vi "Merge Frequency Arrays.vi"(10 "New Frequencies to merge":dbl[](array[numeric]), 11 "Statistics Data":T1) -> (3 "Statistics Data 2":T1)   [LabVIEW 2011]
uses:
  Statistics Data.ctl
  CGI SimpleStat Results.ctl
panel:
  out "Array":dbl[](array[numeric]) format="%_17f"
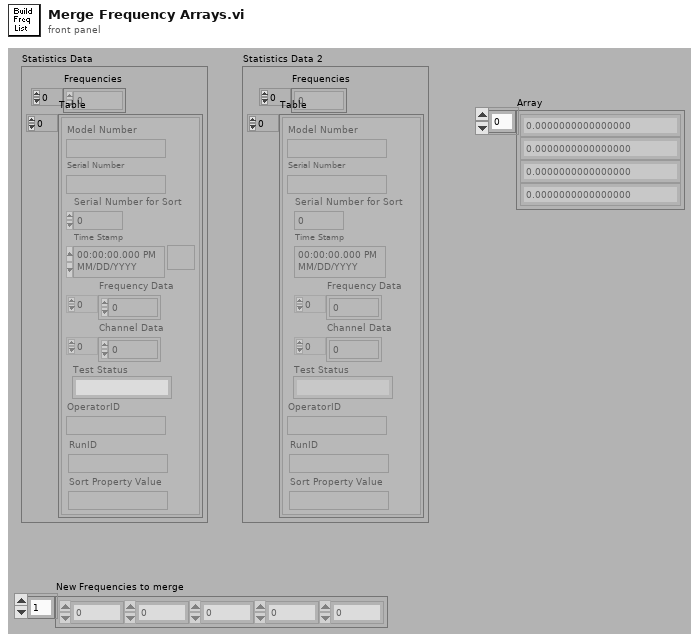
[diagram p1: front panel]
types:
  T1 = typedef "Statistics Data.ctl" = cluster{"Table":T2[], "Frequencies":dbl[]}
  T2 = typedef "CGI SimpleStat Results.ctl" = cluster{"Model Number":string, "Serial Number for Sort":i32, "Serial Number":string, "Time Stamp":timestamp, "Channel Data":dbl[], "Test Status":string, "OperatorID":string, "Frequency Data":dbl[], "RunID":string, "Sort Property Value":string}
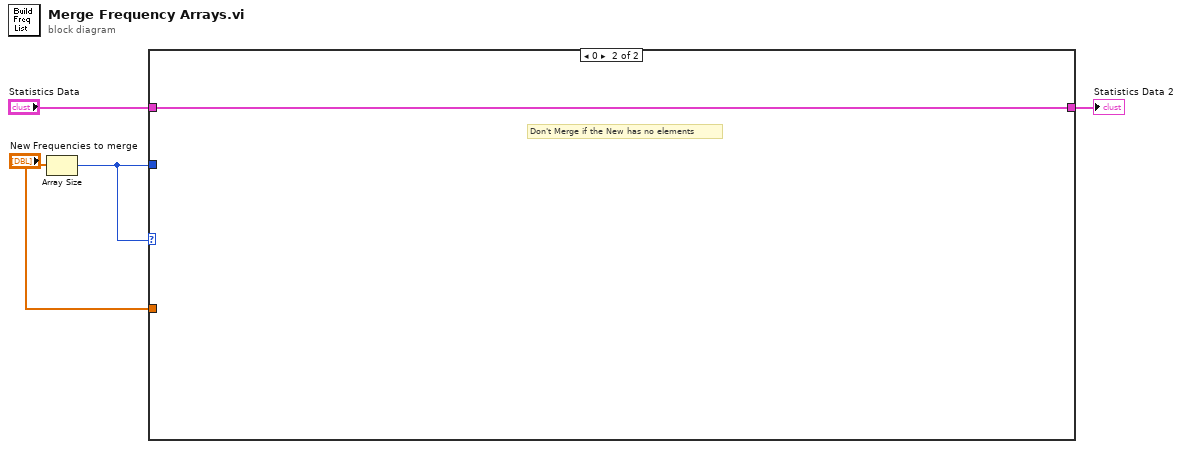
[diagram p0: block diagram]
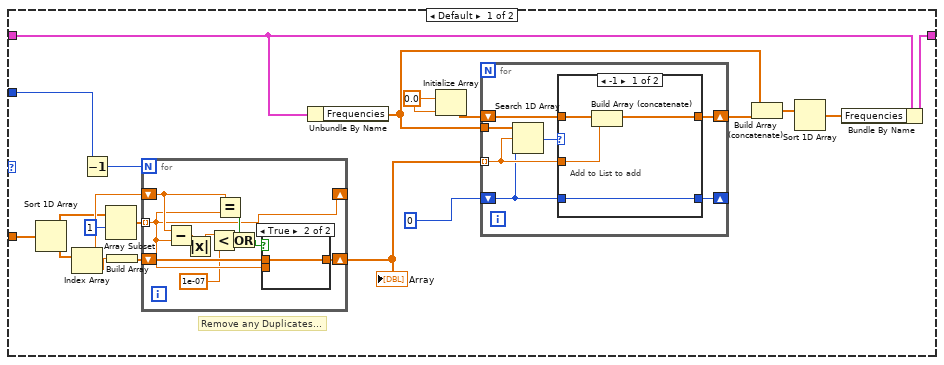
[diagram p2: hidden frame]
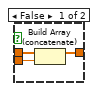
[diagram p3: hidden frame]
diagram:
  n1 = Array Size(array="New Frequencies to merge") -> (size(s)=w1:i32)
  n2 = case shown="0" w1 {
    tunnel: "Statistics Data" -> [w21 w50]
    tunnel: [w20 w50] -> w3
    tunnel: w1 -> [w13 _]
    tunnel: "New Frequencies to merge" -> [w10 _]
    frame Default {
      w17 = 0.0
      # "Remove any Duplicates..."
      n3 = Sort 1D Array(array=w10) -> (sorted array=w5:dbl[])
      n4 = Index Array(array=w5) -> (element=w7:dbl)  [unwired: 1 in]
      n5 = Decrement(x=w13) -> (x-1=w12:i32)
      n6 = Array Subset(array=w5, index=1) -> (w8:dbl[])  [unwired: 1 in]
      n7 = Build Array(w7) -> (w11:dbl[])
      n8 = for {
        N: w12 -> [_]
        shift-right: [w31] -> w6
        shift-left: w11 -> [w32]
        tunnel: w8 -> [w27] mode=indexing
        shift-right: [w27] -> _
        shift-left: w7 -> [w28]
        n9 = Subtract(x=w28, y=w27) -> (x-y=w24:dbl)
        n10 = Absolute Value(x=w24) -> (abs(x)=w23:dbl)
        n11 = Less?(x=w23, y=1e-07) -> (x < y?=w25:bool)
        n12 = Equal?(x=w28, y=w27) -> (x = y?=w30:bool)
        n13 = Or(x=w30, y=w25) -> (x .or. y?=w29:bool)
        n14 = case shown="True" w29 {
          tunnel: w32 -> [w35 w36]
          tunnel: [w33 w36] -> w31
          tunnel: w27 -> [w34 _]
          frame False {
            n15 = Build Array (concatenate)(w35, w34) -> (w33:dbl[])
          }
          frame True {
          }
        }
      }
      "Array" <- w6
      n16 = Unbundle By Name(w21) -> ("Frequencies"=w15:dbl[])
      n17 = Initialize Array(w17, w17) -> (w18:dbl[])
      n18 = for {
        tunnel: w6 -> [w41] mode=indexing
        shift-right: [w43] -> w16
        shift-left: w18 -> [w42]
        shift-right: [w38] -> _
        shift-left: 0 -> [w40]
        tunnel: w15 -> [w37]
        n19 = Search 1D Array(1D array=w37, element=w41, start index (0)=w40) -> (index of element=w39:i32)
        n20 = case shown="-1" w39 {
          tunnel: [w44 w48] -> w38
          tunnel: [w45 w49] -> w43
          tunnel: w42 -> [w47 w49]
          tunnel: w41 -> [w46 _]
          tunnel: w40 -> [w44 w48]
          frame -1 {
            # "Add to List to add"
            n21 = Build Array (concatenate)(w47, w46) -> (w45:dbl[])
          }
          frame Default {
            # "Found this frequency\nDon't add to the list."
          }
        }
      }
      n22 = Build Array (concatenate)(w15, w16) -> (w14:dbl[])
      n23 = Sort 1D Array(array=w14) -> (sorted array=w19:dbl[])
      n24 = Bundle By Name(cluster=w21, "Frequencies"=w19) -> (w20:T1)
    }
    frame 0 {
      # "Don't Merge if the New has no elements"
    }
  }
  "Statistics Data 2" <- w3
